vi "LED Ctlr Cmds.vi"(0 "VISA session":refnum<visa-resource-name>="COM7", 5 "Intensity":dbl(knob) scale=0.0..100.0, 9 "Enable":u8=31, 11 "error in (no error)":errorcluster) -> (4 "VISA session out":refnum<visa-resource-name>, 6 "Bytes at port":u8, 8 "Response":string, 10 "Bytes Read":u8, 15 "error out":errorcluster)   [LabVIEW 2010]
uses:
  <vilib>/Instr/_visa.llb/VISA Configure Serial Port (Instr).vi
panel:
  out "Intensity Set":u16
  in  "Serial Configuration":T1={"Baud Rate"=115200, "Parity"=0, "Data Bits"=8, "Stop Bits"=10, "Flow Control"=0} {"Flow Control" items=["None", "XON/XOFF", "RTS/CTS", "XON/XOFF & RTS/CTS", "DTR/DSR", "XON/XOFF & DTR/DSR"]; "Stop Bits" items=["1.0"=10, "1.5"=15, "2.0"=20]; "Data Bits" items=["7"=7, "8"=8]; "Parity" items=["None", "Odd", "Even", "Mark", "Space"]; "Baud Rate" items=["300"=300, "600"=600, "1200"=1200, "2400"=2400, "4800"=4800, "9600"=9600, "19200"=19200]}
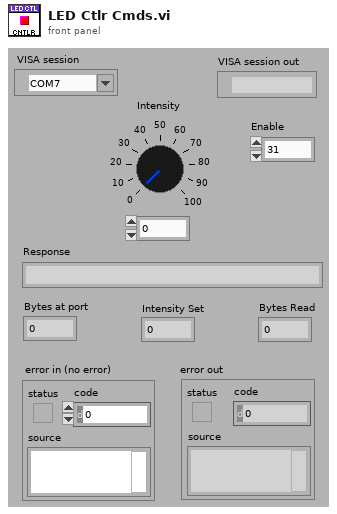
[diagram p1: front panel]
types:
  T1 = cluster{"Baud Rate":u32, "Parity":u16, "Data Bits":u16, "Stop Bits":u16, "Flow Control":u16}
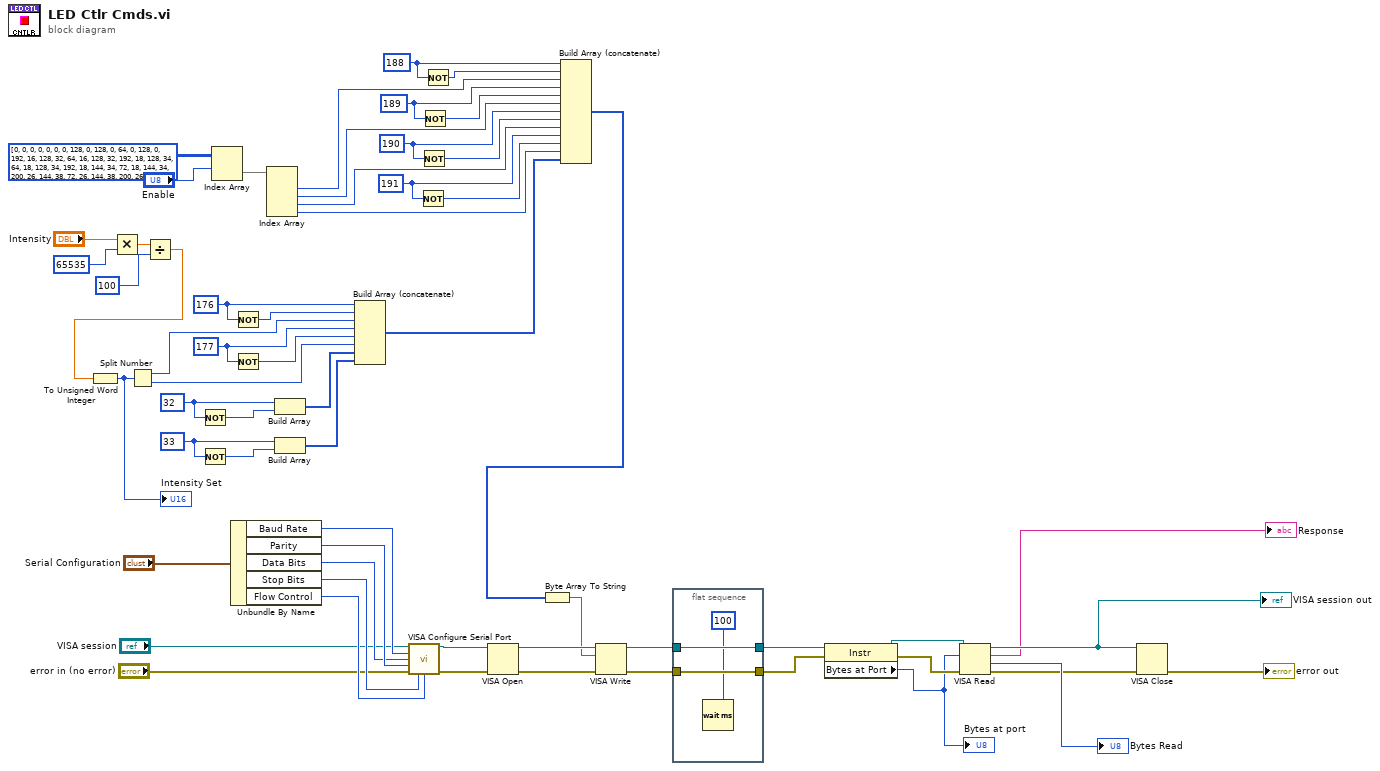
[diagram p0: block diagram]
diagram:
  w10 = u8 33
  w14 = u8 32
  w18 = u8 177
  w21 = u8 176
  w25 = u8 191
  w27 = u8 190
  w30 = u8 189
  w34 = u8 188
  n1 = Multiply(x="Intensity", y=65535) -> (x*y=w4:dbl)
  n2 = Divide(x=w4, y=100) -> (x/y=w2:dbl)
  n3 = To Unsigned Word Integer(number=w2) -> (unsigned 16bit integer=w1:u16)
  "Intensity Set" <- w1
  n4 = Split Number(x=w1) -> (hi(x)=w19:u8, lo(x)=w16:u8)
  n5 = Not(x=w14) -> (.not. x?=w13:u8)
  n6 = Not(x=w10) -> (.not. x?=w11:u8)
  n7 = Index Array(array=u8[][] [[0, 0, 0, 0], [0, 0, 0, 128], [0, 128, 0, 64], [0, 128, 0, 192], [16, 128, 32, 64], [16, 128, 32, 192], [18, 128, 34, 64], [18, 128, 34, 192], [18, 144, 34, 72], [18, 144, 34, 200], [26, 144, 38, 72], [26, 144, 38, 200], [26, 208, 38, 88], [26, 208, 38, 216], [26, 216, 38, 92], [26, 216, 38, 220], [90, 216, 54, 92], [90, 216, 54, 220], [91, 216, 55, 92], [91, 216, 55, 220], [91, 218, 55, 93], [91, 218, 55, 221], [219, 218, 119, 93], [219, 218, 119, 221], [219, 222, 119, 95], [219, 222, 119, 223], [251, 222, 247, 95], [251, 222, 247, 223], [251, 254, 247, 127], [251, 254, 247, 255], [255, 254, 255, 127], [255, 255, 255, 255]], index (row)="Enable") -> (element=w32:u8[])  [unwired: 1 in]
  n8 = Unbundle By Name("Serial Configuration") -> ("Baud Rate"=w59:u32, "Parity"=w58:u16, "Data Bits"=w57:u16, "Stop Bits"=w56:u16, "Flow Control"=w55:u16)
  n9 = Not(x=w21) -> (.not. x?=w20:u8)
  n10 = Not(x=w18) -> (.not. x?=w17:u8)
  n11 = Index Array(array=w32) -> (element #1=w31:u8, element #2=w28:u8, element #3=w23:u8, element #4=w22:u8)  [unwired: 4 in]
  n12 = Build Array(w14, w13) -> (w12:u8[])
  n13 = Build Array(w10, w11) -> (w9:u8[])
  n14 = Build Array (concatenate)(w21, w20, w19, w18, w17, w16, w12, w9) -> (w8:u8[])
  n15 = call-poly "VISA Configure Serial Port"("VISA resource name"="VISA session", "baud rate (9600)"=w59, "data bits (8)"=w57, "parity (0:none)"=w58, "error in (no error)"="error in (no error)", "stop bits (10: 1 bit)"=w56, "flow control (0:none)"=w55) -> ("VISA resource name out"=w52:refnum<visa-resource-name>, "error out"=w51:errorcluster)  [unwired: 7 in]
  n16 = Not(x=w25) -> (.not. x?=w24:u8)
  n17 = Not(x=w27) -> (.not. x?=w26:u8)
  n18 = Not(x=w30) -> (.not. x?=w29:u8)
  n19 = Not(x=w34) -> (.not. x?=w33:u8)
  n20 = VISA Open(error in (no error)=w51, VISA resource name=w52) -> (VISA resource name=w50:refnum<visa-resource-name>, error out=w49:errorcluster)  [unwired: 3 in]
  n21 = Build Array (concatenate)(w34, w33, w31, w30, w29, w28, w27, w26, w23, w25, w24, w22, w8) -> (w7:u8[])
  n22 = Byte Array To String(unsigned byte array=w7) -> (string=w15:string)
  n23 = VISA Write(VISA resource name=w50, write buffer=w15, error in (no error)=w49) -> (VISA resource name out=w47:refnum<visa-resource-name>, error out=w48:errorcluster)  [unwired: 1 out]
  n24 = flat-sequence {
    tunnel: [w63] -> w46
    tunnel: w47 -> [w63]
    tunnel: [w62] -> w45
    tunnel: w48 -> [w62]
    frame #0 {
      n25 = Wait (ms)(milliseconds to wait=100) -> ()  [unwired: 1 out]
    }
  }
  n26 = property class="Instr"(reference=w46, error in=w45) -> (reference out=w44:refnum<visa-resource-name>, error out=w43:errorcluster, "Bytes at Port"=w42:u32)
  "Bytes at port" <- w42
  n27 = VISA Read(VISA resource name=w44, byte count=w42, error in (no error)=w43) -> (VISA resource name out=w39:refnum<visa-resource-name>, read buffer=→"Response":string, return count=→"Bytes Read":u32, error out=w40:errorcluster)
  "VISA session out" <- w39
  n28 = VISA Close(VISA resource name=w39, error in (no error)=w40) -> (error out=→"error out":errorcluster)
